vi "Accuracy Parameter Query.vi"(8 "error in (no error)":errorcluster, 11 "VISA resource name":refnum<visa-resource-name>) -> (0 "error out":errorcluster, 1 "Time Integration":u8, 2 "Voltage Level":dbl format="%.2f", 3 "VISA resource name out":refnum<visa-resource-name>, 5 "Cable Length":i16, 7 "Frequency":dbl format="%.2f")   [LabVIEW 2015, in "Agilent 428X Series.lvlib"]
doc: "This Vi will set a couples of query to obtain the following measurement from the device: voltage level, frequency, cable length, and time integration."
uses:
  <instrlib>/Agilent 428X Series/Agilent 428X Series.lvlib
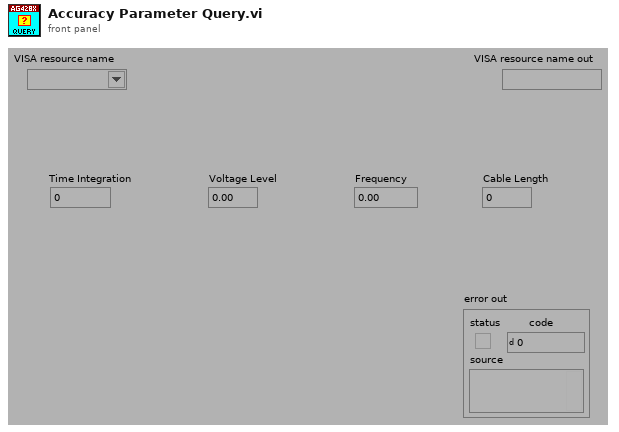
[diagram p1: front panel]
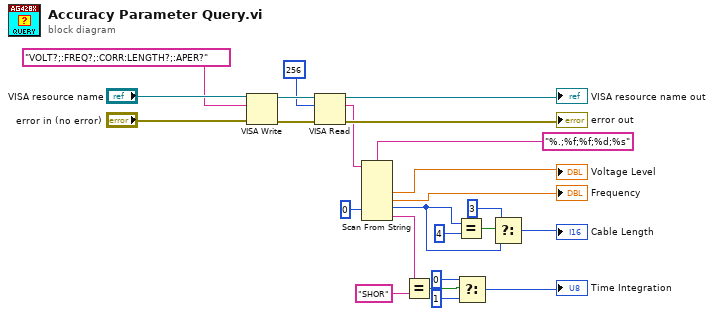
[diagram p0: block diagram]
diagram:
  n1 = VISA Write(VISA resource name="VISA resource name", write buffer="VOLT?;:FREQ?;:CORR:LENGTH?;:APER?" ("write buffer (\"\")"), error in (no error)="error in (no error)") -> (VISA resource name out=w21:refnum<visa-resource-name>, error out=w20:errorcluster)  [unwired: 1 out]
  n2 = VISA Read(VISA resource name=w21, byte count=u32 256 ("byte count (0)"), error in (no error)=w20) -> (VISA resource name out=→"VISA resource name out":refnum<visa-resource-name>, read buffer=w16:string, error out=→"error out":errorcluster)  [unwired: 1 out]
  n3 = Scan From String(format string="%.;%f;%f;%d;%s", input string=w16, default 3=i16 0) -> (output 1=→"Voltage Level":dbl, output 2=→"Frequency":dbl, output 3=w1:i16, output 4=w11:string)  [unwired: 5 in, 3 out]
  n4 = Equal?(x=w11, y="SHOR") -> (x = y?=w9:bool)
  n5 = Equal?(x=w1, y=i16 4) -> (x = y?=w4:bool)
  n6 = Select(t=u8 0, s=w9, f=u8 1) -> (s? t:f=→"Time Integration":u8)
  n7 = Select(t=i16 3 ("f"), s=w4, f=w1) -> (s? t:f=→"Cable Length":i16)
